vi "checkSettled.vi"(8 "error in (no error)":errorcluster, 11 "SystemController in":refnum<class "SystemController.lvclass">) -> (0 "error out":errorcluster, 3 "SystemController out":refnum<class "SystemController.lvclass">)   [LabVIEW 2015]
uses:
  SystemController.lvclass
panel:
  out "settledIsTrue":bool
  in  "resetIsTrue":bool
  in  "Distance Measured":dbl[unit]=1.0 min=1.0 max=300.0 format="%.1f"
  in  "loopPeriod":dbl[unit]=5000.0 min=10.0 max=5000.0
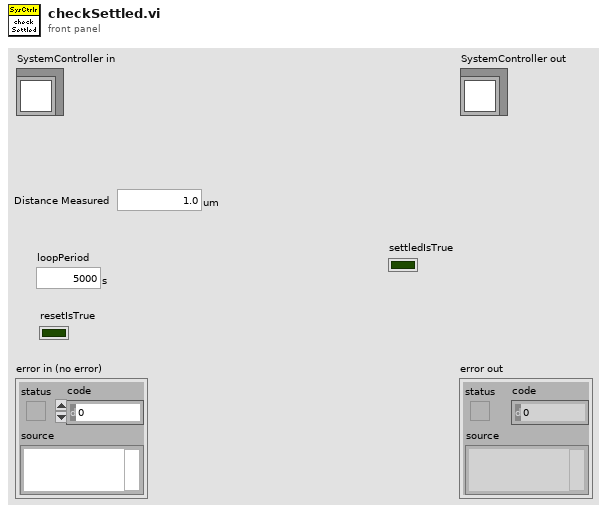
[diagram p1: front panel]
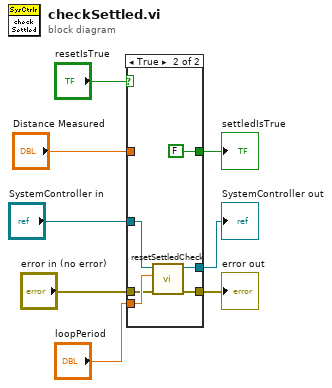
[diagram p0: block diagram]
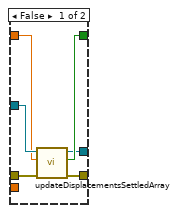
[diagram p2: hidden frame]
diagram:
  n1 = case shown="True" "resetIsTrue" {
    tunnel: [w14 FALSE ("settledIsTrue")] -> w8
    tunnel: "SystemController in" -> [w13 w20]
    tunnel: [w12 w19] -> w5
    tunnel: "Distance Measured" -> [w11 _]
    tunnel: "loopPeriod" -> [_ w17]
    tunnel: "error in (no error)" -> [w10 w16]
    tunnel: [w9 w15] -> w1
    frame False {
      n2 = call "updateDisplacementsSettledArray.vi"("error in (no error)"=w10, "Distance Measured"=w11, "SystemController in"=w13) -> ("error out"=w9:errorcluster, "settledIsTrue"=w14:bool, "SystemController out"=w12:refnum<class "SystemController.lvclass">)  [unwired: 6 in]
    }
    frame True {
      n3 = call "resetSettledCheck.vi"("error in (no error)"=w16, "loopPeriod"=w17, "SystemController in"=w20) -> ("error out"=w15:errorcluster, "SystemController out"=w19:refnum<class "SystemController.lvclass">)  [unwired: 6 in, 1 out]
    }
  }
  "error out" <- w1
  "SystemController out" <- w5
  "settledIsTrue" <- w8
